vi "QPSK Modulation(SubVI).vi"(10 "standard deviation":dbl=1.0000000000000002 format="%0.2f", 11 "Sequence Size":i32) -> (1 "Transmitted Signal":waveform(dbl)(graph), 2 "input bits":dbl[](array[numeric]), 3 "Input Graph":dbl[](graph), 4 "Array":dynamicdata[](array[waveform]), 5 "size(s)":i32)   [LabVIEW 2026]
uses:
  <vilib>/Waveform/WDTOps.llb/WDT Append Waveforms DBL.vi
  <vilib>/Analysis/NI_AALBase.lvlib
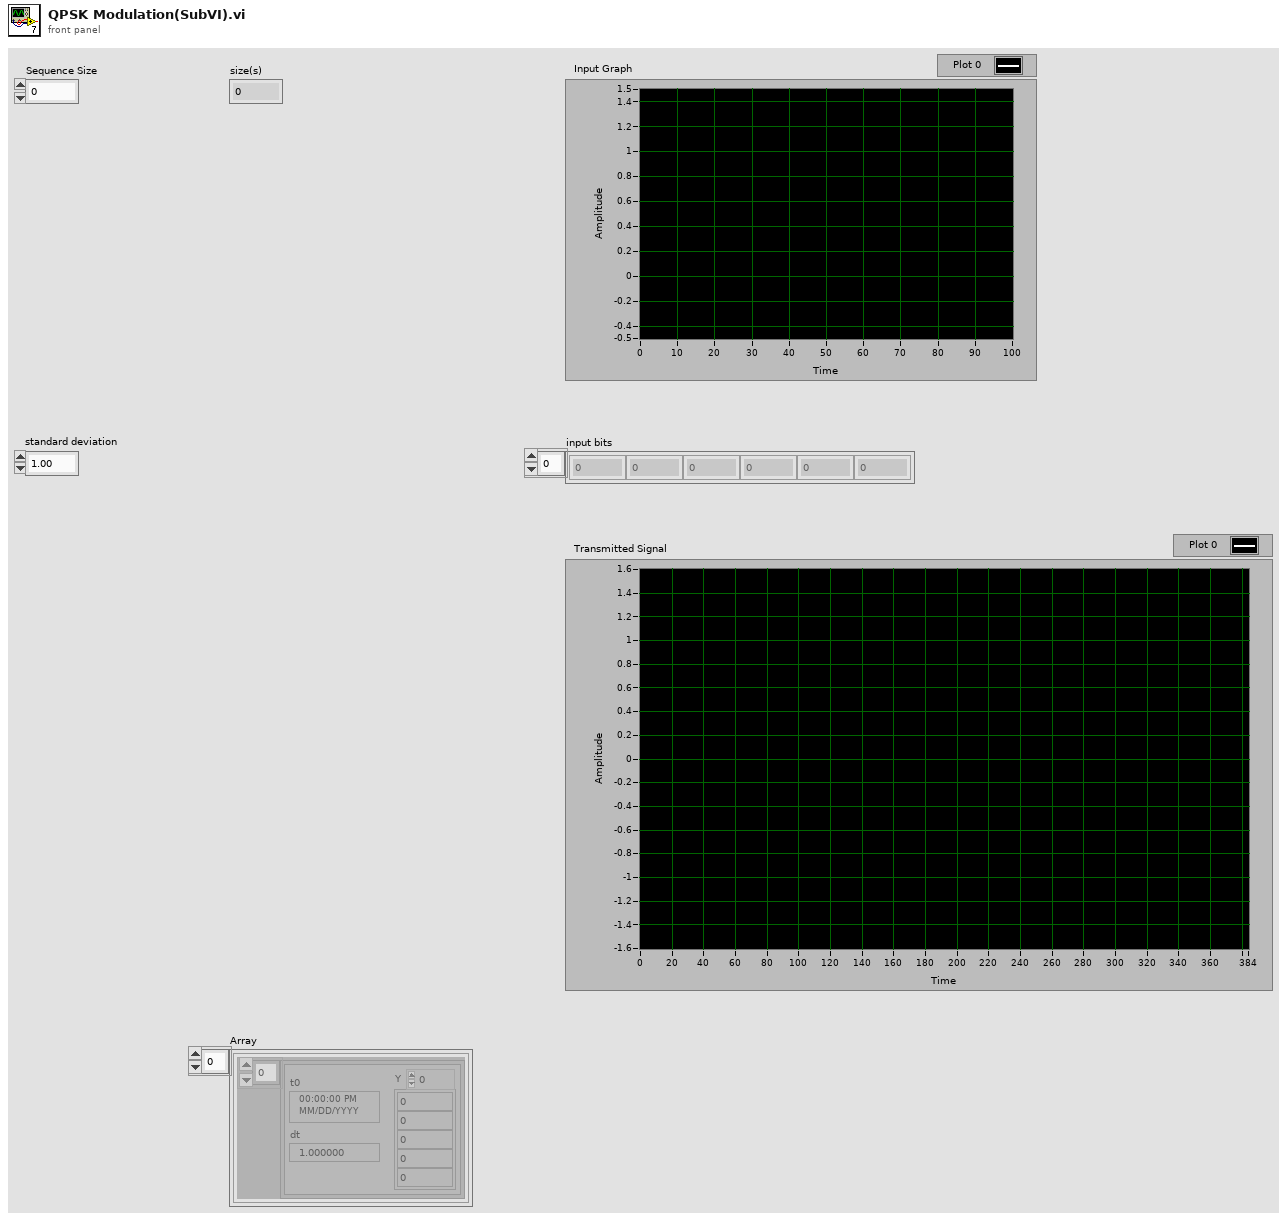
[diagram p1: front panel]
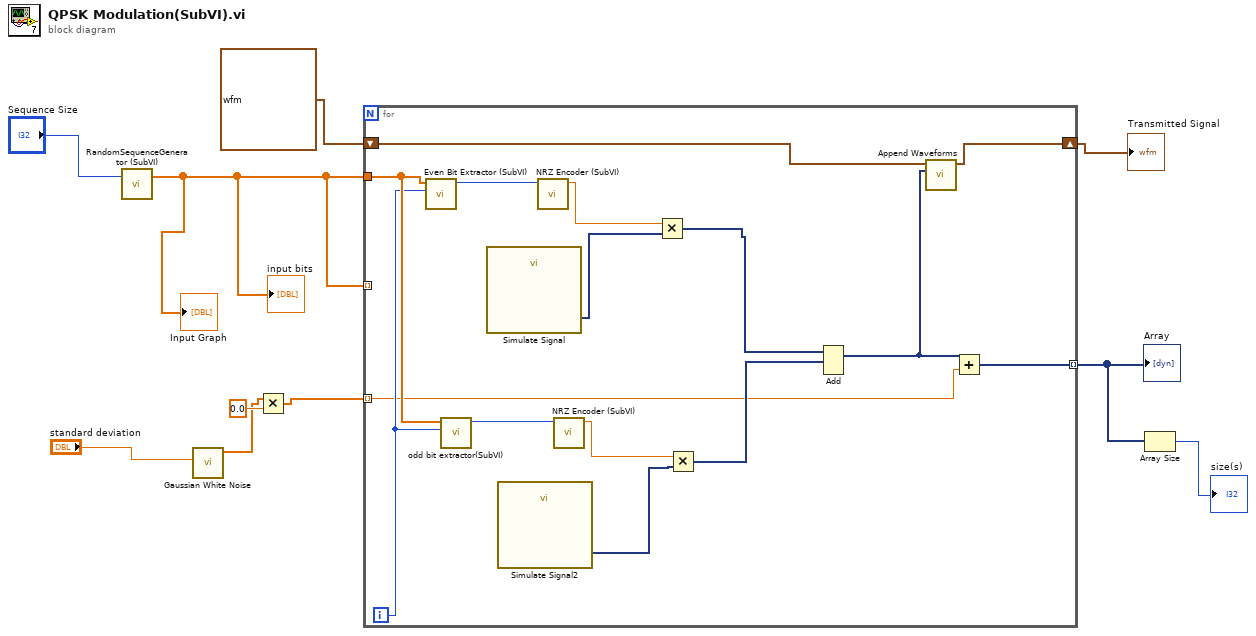
[diagram p0: block diagram]
diagram:
  n1 = call "RandomSequenceGenerator (SubVI).vi"("Numeric"="Sequence Size") -> ("Array"=w8:dbl[])  [unwired: 1 in, 1 out]
  "input bits" <- w8
  "Input Graph" <- w8
  n2 = call <vilib>:"Gaussian White Noise.vi"("standard deviation"="standard deviation") -> ("Gaussian noise pattern"=w2:dbl[])  [unwired: 9 in, 1 out]
  n3 = Multiply(x=w2, y=0.0) -> (x*y=w1:dbl[])
  n4 = for {
    tunnel: w8 -> [w25]
    tunnel: [w11] -> w9 mode=indexing
    tunnel: w1 -> [w15] mode=indexing
    shift-right: [w12] -> w7
    shift-left: waveform(dbl) {"t0"=timestamp(0 s since 1904-01-01), "dt"=1.0, "Y"=[]} ("Waveform") -> [w13]
    tunnel: w8 -> [_] mode=indexing
    i -> [w24]
    n5 = call "Even Bit Extractor (SubVI).vi"("loop Index"=w24, "Input PN sequence"=w25) -> ("Even Bits"=w23:i8)  [unwired: 9 in]
    n6 = call "odd bit extractor(SubVI).vi"("Loop Index"=w24, "input PN Sequence"=w25) -> ("Odd bits"=w22:i8)  [unwired: 9 in]
    n7 = call "Simulate Signal"() -> ("Cosine"=w21:dynamicdata)  [unwired: 14 in, 1 out]
    n8 = call "Simulate Signal2"() -> ("Sine"=w18:dynamicdata)  [unwired: 14 in, 1 out]
    n9 = call "NRZ Encoder (SubVI).vi"("Input Bit"=w23) -> ("NRZ Output"=w20:dbl)  [unwired: 10 in]
    n10 = call "NRZ Encoder (SubVI).vi"("Input Bit"=w22) -> ("NRZ Output"=w19:dbl)  [unwired: 10 in]
    n11 = Multiply(x=w20, y=w21) -> (x*y=w17:dynamicdata)
    n12 = Multiply(x=w19, y=w18) -> (x*y=w16:dynamicdata)
    n13 = Add(1:w16, 2:w17) -> (0:w14:dynamicdata)  [unwired: 1 in, 1 out]
    n14 = call-poly <vilib>:"Append Waveforms.vi"("waveform B"=w14, "waveform A"=w13) -> ("waveform out"=w12:waveform(dbl))  [unwired: 8 in, 1 out]
    n15 = Add(x=w14, y=w15) -> (x+y=w11:dynamicdata)
  }
  "Transmitted Signal" <- w7
  "Array" <- w9
  n16 = Array Size(array=w9) -> (size(s)=→"size(s)":i32)
